vi "setup_window.vi"() -> ()   [LabVIEW 2017]
doc: "the window displazs the main setup data"
uses:
  global variables.vi
  Classes/StatusLog/StatusLog.lvclass
panel:
  in  "Tab Control":T1(tab)
  in  "logfile":path
  in  "Instruments Listbox":i32(listbox)
  in  "SysChkDev Listbox":i32(listbox)
  in  "Switches Listbox":i32(listbox)
  in  "Standards Tree":string(tree)
  in  "Menu Listbox":i32(listbox)
  # "General settings"
  # "List of all instruments and their settings"
  # "List of all system check devices such as pressure and temperature sensors"
  # "List of all switches and their settings"
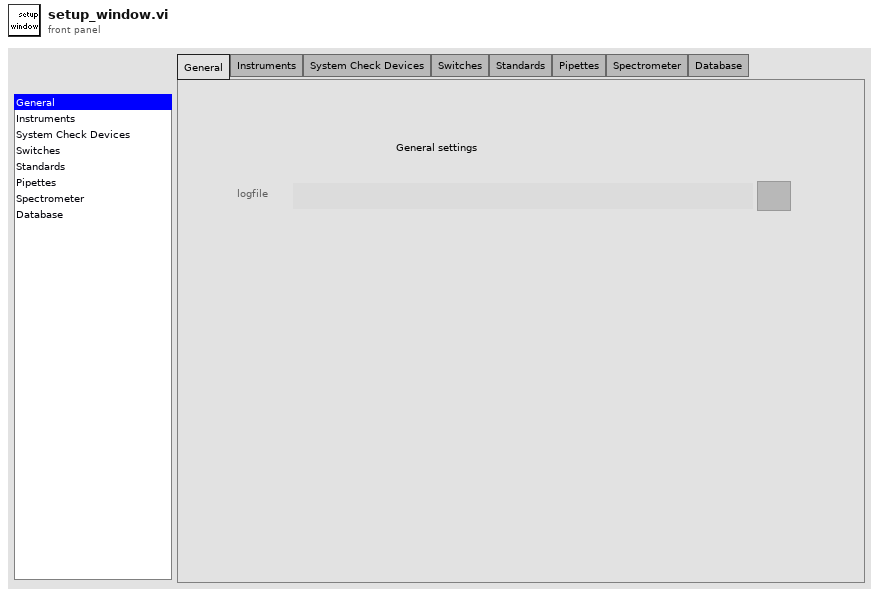
[diagram p1: front panel]
types:
  T1 = enum32{"General", "Instruments", "System Check Devices", "Switches", "Standards", "Pipettes", "Spectrometer", "Database"}
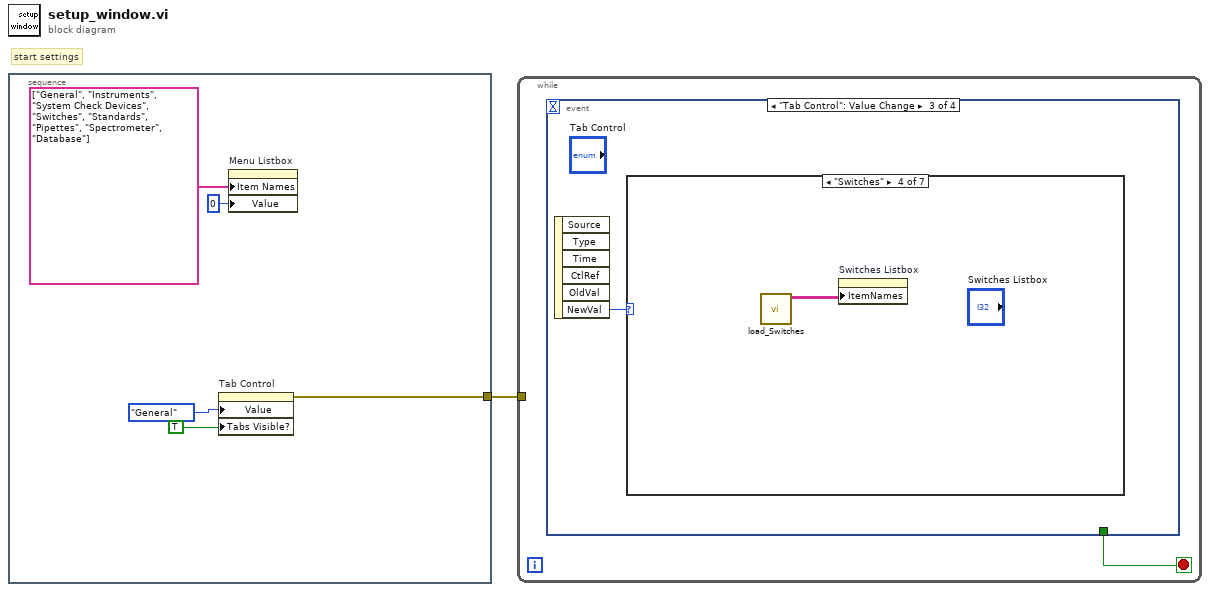
[diagram p0: block diagram]
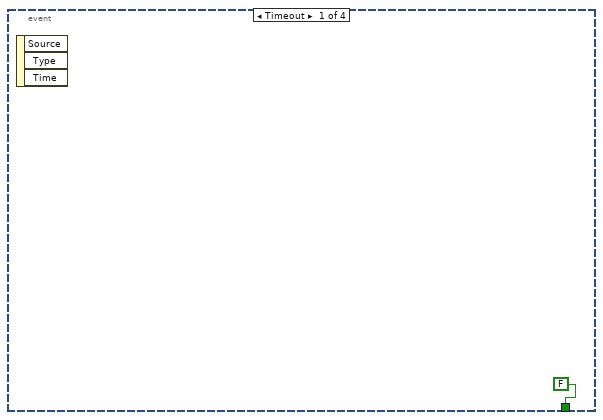
[diagram p2: hidden frame]
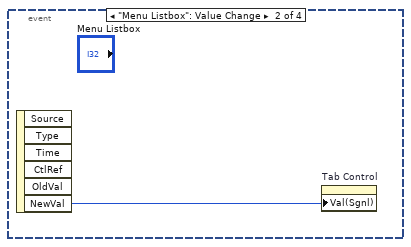
[diagram p3: hidden frame]
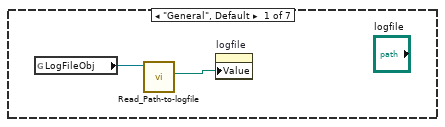
[diagram p4: hidden frame]
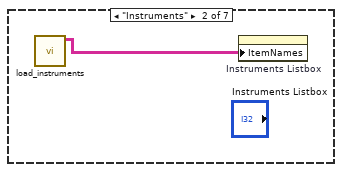
[diagram p5: hidden frame]
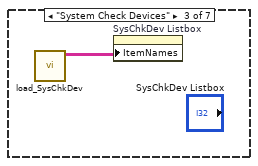
[diagram p6: hidden frame]
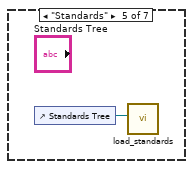
[diagram p7: hidden frame]
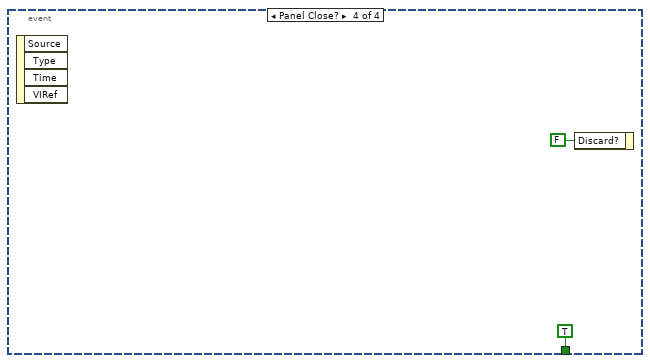
[diagram p10: hidden frame]
diagram:
  # "start settings"
  n1 = stacked-sequence {
    tunnel: [w2] -> w1
    frame #0 {
      n2 = property on="Tab Control" class="TabCtl (strict)"("Value"=T1."General" ("Tab Control"), "Tabs Visible?"=TRUE) -> (error out=w2:errorcluster)  [unwired: 2 in, 1 out]
      n3 = property on="Menu Listbox" class="LstBox (strict)"("Item Names"=string[] ["General", "Instruments", "System Check Devices", "Switches", "Standards", "Pipettes", "Spectrometer", "Database"], "Value"=0 ("Menu Listbox")) -> ()  [unwired: 2 in, 2 out]
    }
  }
  n4 = while {
    tunnel: w1 -> [_]
    stop <- w7 stop-if-true
    n5 = event shown="[2] \"Tab Control\": Value Change" {
      selector: _ -> [_ _ _ _]
      dyn-events: _ -> [_ _ _ _]
      timeout: _ -> [_ _ _ _]
      tunnel: [FALSE _ _ TRUE] -> w7
      event Timeout {
        n6 = event-data() -> ()  [unwired: 1 in, 3 out]
      }
      event "Menu Listbox": Value Change {
        n7 = event-data() -> ("NewVal"=w9:i32)  [unwired: 1 in, 5 out]
        n8 = property on="Tab Control" class="TabCtl (strict)"("Val(Sgnl)"=w9) -> ()  [unwired: 2 in, 2 out]
      }
      event "Tab Control": Value Change {
        n9 = event-data() -> ("NewVal"=w10:T1)  [unwired: 1 in, 5 out]
        n10 = case shown="\"Switches\"" w10 {
          frame "General", Default {
            n11 = global read "global variables.vi" "LogFileObj"() -> (w12:refnum<class "StatusLog.lvclass">)
            n12 = call-dynamic "Read_Path-to-logfile.vi"("StatusLog in"=w12) -> ("Path to logfile"=w11:path)  [unwired: 8 in, 2 out]
            n13 = property on="logfile" class="Path"("Value"=w11) -> ()  [unwired: 2 in, 2 out]
          }
          frame "Instruments" {
            n14 = call "load_instruments.vi"() -> ("output array"=w13:string[][])  [unwired: 11 in]
            n15 = property on="Instruments Listbox" class="MCListbox (strict)"("ItemNames"=w13) -> ()  [unwired: 2 in, 2 out]
          }
          frame "System Check Devices" {
            n16 = call "load_SysChkDev.vi"() -> ("output array"=w14:string[][])  [unwired: 11 in]
            n17 = property on="SysChkDev Listbox" class="MCListbox (strict)"("ItemNames"=w14) -> ()  [unwired: 2 in, 2 out]
          }
          frame "Switches" {
            n18 = call "load_Switches.vi"() -> ("output array"=w15:string[][])  [unwired: 11 in]
            n19 = property on="Switches Listbox" class="MCListbox (strict)"("ItemNames"=w15) -> ()  [unwired: 2 in, 2 out]
          }
          frame "Standards" {
            n20 = control-ref of="Standards Tree"() -> (w16:refnum<vi>)
            n21 = call "load_standards.vi"("Standards Tree ref"=w16) -> ()  [unwired: 11 in]
          }
          frame "Pipettes" {
          }
          frame "Spectrometer" {
          }
        }
      }
      event Panel Close? {
        n22 = event-data() -> ()  [unwired: 1 in, 4 out]
        n23 = event-data("Discard?"=FALSE) -> ()  [unwired: 1 in, 1 out]
      }
    }
  }
